vi "Save Project.vi"(8 "error in (no error)":errorcluster, 10 "Save As":bool, 11 "Editor.lvclass in":refnum<data-value>) -> (0 "error out":errorcluster, 2 "Cancelled":bool caption="cancelled", 3 "Editor.lvclass out":refnum<data-value>)   [LabVIEW 2015, in "Editor.lvclass"]
uses:
  Editor.lvclass
  Project.lvclass
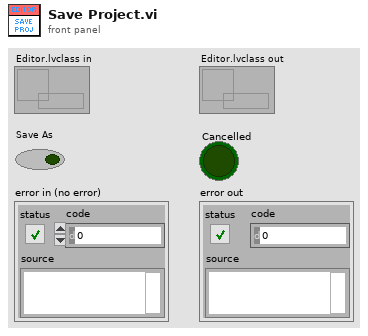
[diagram p1: front panel]
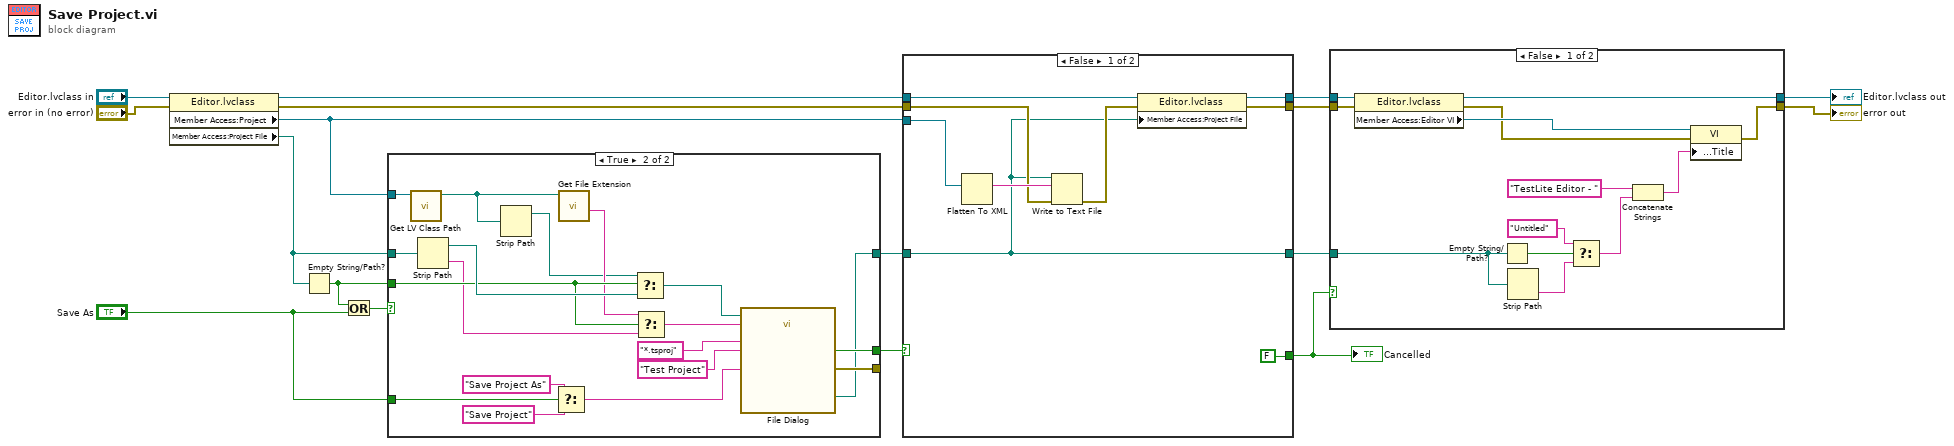
[diagram p0: block diagram]
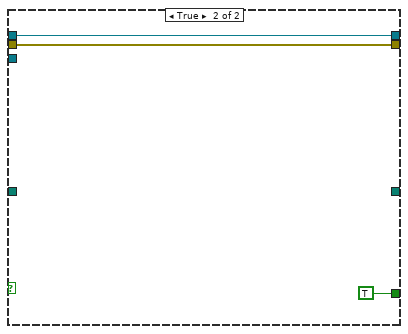
[diagram p3: hidden frame]
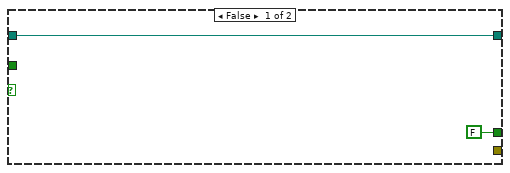
[diagram p4: hidden frame]
diagram:
  n1 = property class="Editor.lvclass"(reference="Editor.lvclass in", error in="error in (no error)") -> (reference out=w8:refnum<data-value>, error out=w9:errorcluster, "Member Access:Project"=w11:refnum<class "Project.lvclass">, "Member Access:Project File"=w14:path)
  n2 = Empty String/Path?(string/path=w14) -> (empty?=w13:bool)
  n3 = Or(x=w13, y="Save As") -> (x .or. y?=w15:bool)
  n4 = case shown="True" w15 {
    tunnel: w14 -> [w19 w36]
    tunnel: w13 -> [_ w33]
    tunnel: w11 -> [_ w22]
    tunnel: [FALSE ("cancelled") w29] -> w12
    tunnel: [_ w28] -> _
    tunnel: [w19 w27] -> w10
    tunnel: "Save As" -> [_ w24]
    frame False {
    }
    frame True {
      n5 = call <vilib>:"Get LV Class Path.vi"("object"=w22) -> ("class path"=w21:path)  [unwired: 9 in, 1 out]
      n6 = Strip Path(path=w36) -> (stripped path=w35:path, name=w32:string)
      n7 = Strip Path(path=w21) -> (stripped path=w20:path)  [unwired: 1 out]
      n8 = Select(t="Save Project As", s=w24, f="Save Project") -> (s? t:f=w23:string)
      n9 = call <vilib>:"Get File Extension.vi"("file"=w21) -> ("filename without extension"=w31:string)  [unwired: 6 in, 4 out]
      n10 = Select(t=w20, s=w33, f=w35) -> (s? t:f=w34:path)
      n11 = Select(t=w31, s=w33, f=w32) -> (s? t:f=w30:string)
      n12 = call "File Dialog"("start path"=w34, "prompt"=w23, "default name"=w30, "pattern (all files)"="*.tsproj" ("pattern label"), "pattern label"="Test Project" ("button label")) -> ("selected path"=w27:path, "cancelled"=w29:bool, "error out"=w28:errorcluster)  [unwired: 7 in, 1 out]
    }
  }
  n13 = case shown="False" w12 {
    tunnel: w11 -> [w46 _]
    tunnel: w10 -> [w39 _]
    tunnel: w9 -> [w45 w50]
    tunnel: w8 -> [w44 w49]
    tunnel: [w42 w49] -> w6
    tunnel: [w41 w50] -> w4
    tunnel: [FALSE TRUE] -> w1
    tunnel: [w39 _] -> w5
    frame False {
      n14 = Flatten To XML(anything=w46) -> (xml string=w47:string)
      n15 = Write to Text File(file (use dialog)=w39, text=w47, error in=w45) -> (error out=w43:errorcluster)  [unwired: 1 in, 2 out]
      n16 = property class="Editor.lvclass"(reference=w44, error in=w43, "Member Access:Project File"=w39) -> (reference out=w42:refnum<data-value>, error out=w41:errorcluster)
    }
    frame True {
    }
  }
  "Cancelled" <- w1
  n17 = case shown="False" w1 {
    tunnel: w6 -> [w57 w65]
    tunnel: w5 -> [w55 _]
    tunnel: w4 -> [w53 w64]
    tunnel: [w52 w65] -> w3
    tunnel: [w51 w64] -> w2
    frame False {
      n18 = property class="Editor.lvclass"(reference=w57, error in=w53) -> (reference out=w52:refnum<data-value>, error out=w54:errorcluster, "Member Access:Editor VI"=w56:refnum<vi>)
      n19 = Empty String/Path?(string/path=w55) -> (empty?=w63:bool)
      n20 = Strip Path(path=w55) -> (name=w62:string)  [unwired: 1 out]
      n21 = Select(t="Untitled", s=w63, f=w62) -> (s? t:f=w59:string)
      n22 = Concatenate Strings("TestLite Editor - ", w59) -> (w58:string)
      n23 = property class="VI"(reference=w56, error in=w54, "Front Panel.Title"=w58) -> (error out=w51:errorcluster)  [unwired: 1 out]
    }
    frame True {
    }
  }
  "Editor.lvclass out" <- w3
  "error out" <- w2
